vi "HexapodMoveHardware.vi"(7 "xyzuvw":dbl[](array[numeric]), 8 "error in (no error)":errorcluster, 9 "Positions of Axes to move":dbl[](array[numeric]), 10 "Axes to move":string[](array[string]), 11 "HexapodPI in":refnum<class "HexapodPI.lvclass">) -> (0 "error out":errorcluster, 2 "Connection":T1, 3 "Move possible":cluster{"status":bool, "message":string})   [LabVIEW 2020, in "HexapodPI.lvclass"]
uses:
  HexapodPI.lvclass
  HexapodPI.lvclass/HexapodPI.ctl
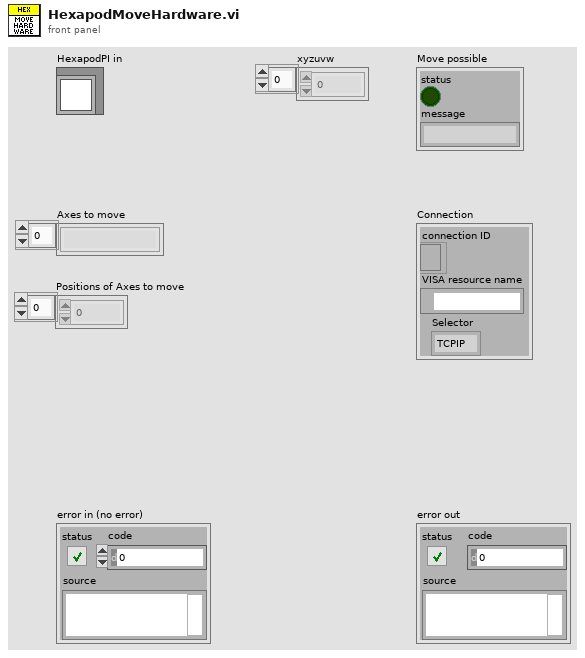
[diagram p1: front panel]
types:
  T1 = cluster{"connection ID":refnum<k5>, "VISA resource name":refnum<visa-resource-name>, "Selector":enum16{"TCPIP", "Serial"}}
  T2 = typedef "OnOffTypeDef.ctl" = enum16{"off", "on"}
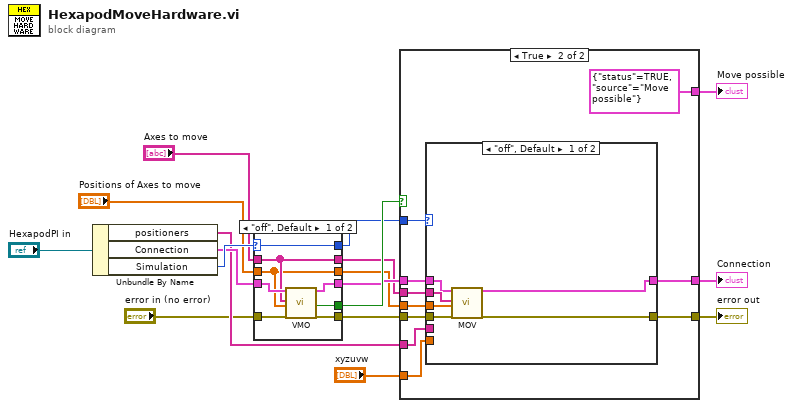
[diagram p0: block diagram]
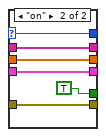
[diagram p2: hidden frame]
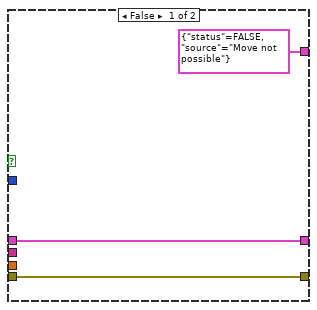
[diagram p3: hidden frame]
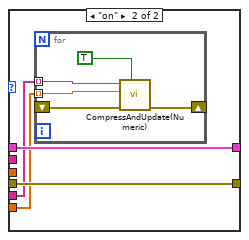
[diagram p4: hidden frame]
diagram:
  n1 = Unbundle By Name("HexapodPI in") -> ("positioners"=w14:string[], "Connection"=w15:T1, "Simulation"=w16:T2)
  n2 = case shown="\"off\", Default" w16 {
    selector: w16 -> [w18 w26]
    tunnel: "error in (no error)" -> [w25 w29]
    tunnel: "Positions of Axes to move" -> [w19 w27]
    tunnel: w15 -> [w24 w31]
    tunnel: "Axes to move" -> [w20 w28]
    tunnel: [w23 w31] -> w8
    tunnel: [w22 w29] -> w9
    tunnel: [w21 TRUE ("Move possible")] -> w11
    tunnel: [w20 w28] -> w3
    tunnel: [w19 w27] -> w2
    tunnel: [w18 w26] -> w1
    frame "off", Default {
      n3 = call "VMO.vi"("Connection"=w24, "Axes to command"=w20, "Position values"=w19, "error in"=w25) -> ("Connection out"=w23:T1, "Move possible"=w21:bool, "error out"=w22:errorcluster)  [unwired: 13 in]
    }
    frame "on" {
    }
  }
  n4 = case shown="True" w11 {
    tunnel: w9 -> [w33 w44]
    tunnel: [w33 w43] -> w5
    tunnel: w3 -> [_ w42]
    tunnel: w2 -> [_ w41]
    tunnel: w8 -> [w34 w40]
    tunnel: [w34 w39] -> w12
    tunnel: [cluster{"status":bool, "source":string} {"status"=FALSE, "source"="Move not possible"} ("error out") cluster{"status":bool, "source":string} {"status"=TRUE, "source"="Move possible"} ("error out")] -> w10
    tunnel: w1 -> [_ w37]
    tunnel: w14 -> [_ w36]
    tunnel: "xyzuvw" -> [_ w35]
    frame False {
    }
    frame True {
      n5 = case shown="\"off\", Default" w37 {
        tunnel: w44 -> [w50 w53]
        tunnel: [w49 w53] -> w43
        tunnel: w42 -> [w48 _]
        tunnel: w41 -> [w47 _]
        tunnel: w40 -> [w46 w54]
        tunnel: [w45 w54] -> w39
        tunnel: w36 -> [_ w52]
        tunnel: w35 -> [_ w51]
        frame "off", Default {
          n6 = call "MOV.vi"("Connection"=w46, "Axes to move"=w48, "Position values"=w47, "error in"=w50) -> ("Connection out"=w45:T1, "error out"=w49:errorcluster)  [unwired: 14 in]
        }
        frame "on" {
          n7 = for {
            tunnel: w52 -> [w56] mode=indexing
            shift-right: [w59] -> _
            shift-left: _ -> [w57]
            tunnel: w51 -> [w55] mode=indexing
            n8 = call "CompressAndUpdate(Numeric).vi"("force CVT update (false)"=TRUE, "error in"=w57, "Numeric"=w55, "command or variable name"=w56) -> ("error out"=w59:errorcluster)  [unwired: 7 in]
          }
        }
      }
    }
  }
  "Connection" <- w12
  "Move possible" <- w10
  "error out" <- w5
